vi "gnuplot_legend.vi"(1 "Plot style":i32[](array[numeric])=[1, 3, 6, 2, 4, 7, 5, 8], 2 "Legend":string[](array[string])) -> (0 "Tex String":string)   [LabVIEW 2010]
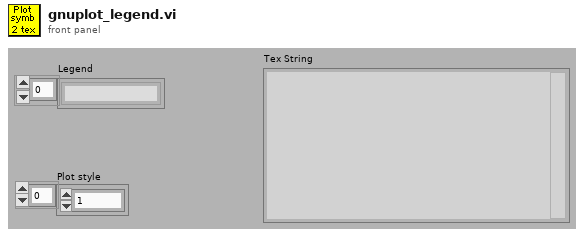
[diagram p1: front panel]
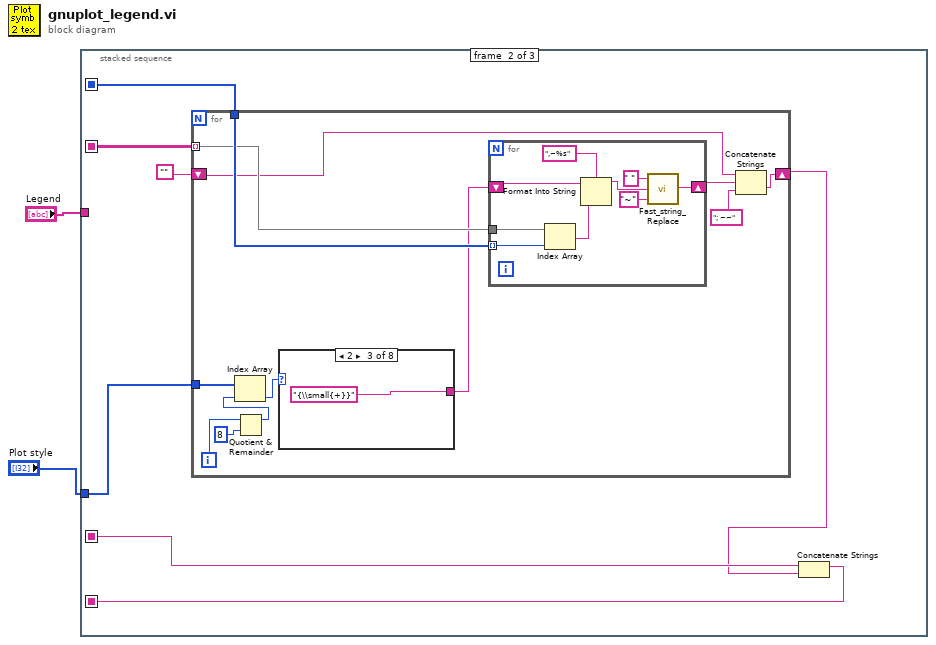
[diagram p0: block diagram]
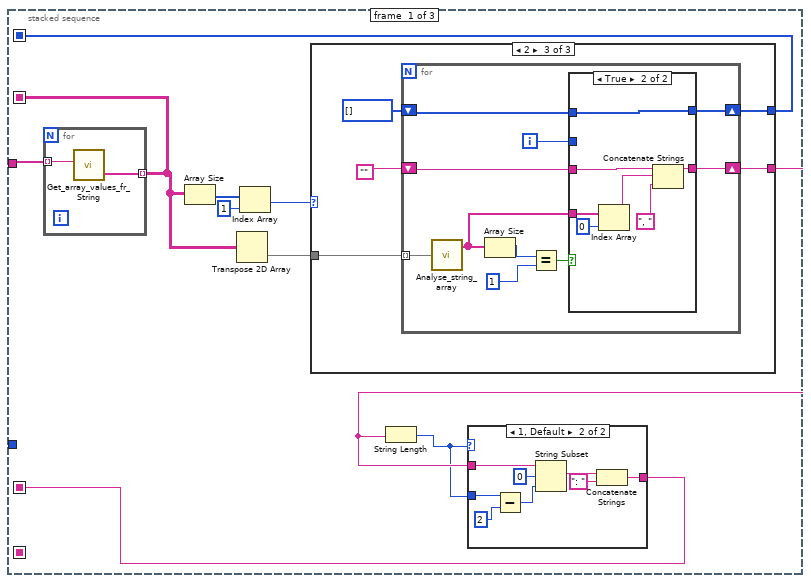
[diagram p2: hidden frame]
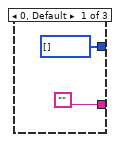
[diagram p4: hidden frame]
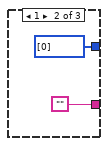
[diagram p5: hidden frame]
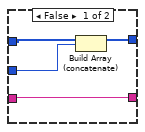
[diagram p6: hidden frame]
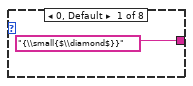
[diagram p7: hidden frame]
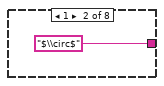
[diagram p8: hidden frame]
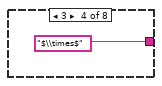
[diagram p9: hidden frame]
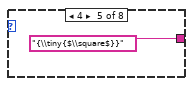
[diagram p10: hidden frame]
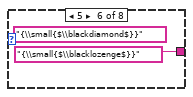
[diagram p11: hidden frame]
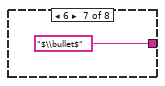
[diagram p12: hidden frame]
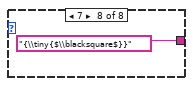
[diagram p13: hidden frame]
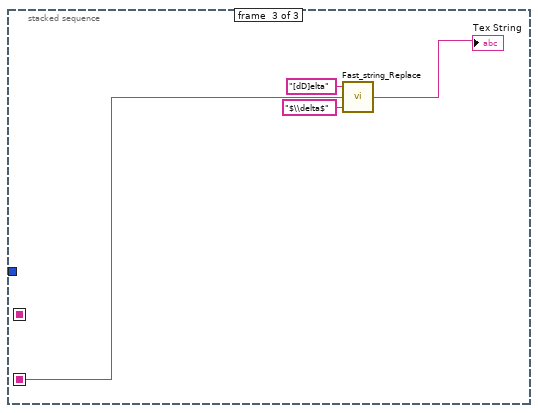
[diagram p14: hidden frame]
diagram:
  n1 = stacked-sequence {
    seq-local: [w8 _ _] -> [_ w60 _]
    seq-local: [w3 _ _] -> [_ w57 _]
    seq-local: [w7 _ _] -> [_ w59 _]
    seq-local: [_ w55 _] -> [_ _ w92]
    tunnel: "Legend" -> [w12 _ _]
    tunnel: "Plot style" -> [_ w54 _]
    frame #0 {
      n2 = for {
        tunnel: w12 -> [w53] mode=indexing
        tunnel: [w52] -> w7 mode=indexing
        n3 = call "Get_array_values_fr_String.vi"("String Value"=w53) -> ("String array"=w52:string[])  [unwired: 1 out]
      }
      n4 = Array Size(array=w7) -> (size(s)=w11:i32[])
      n5 = Transpose 2D Array(2D array=w7) -> (transposed array=w9:string[][])
      n6 = Index Array(array=w11, index=1) -> (element=w6:i32)
      n7 = case shown="2" w6 {
        tunnel: w9 -> [_ _ w30]
        tunnel: [i32[] [] i32[] [0] w28] -> w8
        tunnel: ["" "" w27] -> w5
        frame 0, Default {
        }
        frame 1 {
        }
        frame 2 {
          n8 = for {
            tunnel: w30 -> [w40] mode=indexing
            shift-right: [w34] -> w27
            shift-left: "" -> [w35]
            shift-right: [w32] -> w28
            shift-left: i32[] [] -> [w33]
            i -> [w31]
            n9 = call "Analyse_string_array.vi"("String array"=w40) -> ("Unique strings"=w36:string[])  [unwired: 2 out]
            n10 = Array Size(array=w36) -> (size(s)=w39:i32)
            n11 = Equal?(x=w39, y=1) -> (x = y?=w37:bool)
            n12 = case shown="True" w37 {
              tunnel: w36 -> [_ w51]
              tunnel: w35 -> [w41 w48]
              tunnel: [w41 w47] -> w34
              tunnel: w33 -> [w43 w46]
              tunnel: [w42 w46] -> w32
              tunnel: w31 -> [w44 _]
              frame False {
                n13 = Build Array (concatenate)(w43, w44) -> (w42:i32[])
              }
              frame True {
                n14 = Index Array(array=w51, index=0) -> (element=w49:string)
                n15 = Concatenate Strings(w48, w49, ", " ("string")) -> (w47:string)
              }
            }
          }
        }
      }
      n16 = String Length(string=w5) -> (length=w4:i32)
      n17 = case shown="1, Default" w4 {
        tunnel: w5 -> [w13 w20]
        tunnel: w4 -> [_ w16]
        tunnel: [w13 w17] -> w3
        frame 0 {
        }
        frame 1, Default {
          n18 = Subtract(x=w16, y=2) -> (x-y=w15:i32)
          n19 = String Subset(string=w20, offset (0)=0, length (rest)=w15) -> (substring=w19:string)
          n20 = Concatenate Strings(w19, ": " ("string")) -> (w17:string)
        }
      }
    }
    frame #1 {
      n21 = for {
        tunnel: w60 -> [w72]
        tunnel: w59 -> [w71] mode=indexing
        shift-right: [w69] -> w56
        shift-left: "" -> [w66]
        tunnel: w54 -> [w61]
        i -> [w65]
        n22 = Quotient & Remainder(x=w65, y=8) -> (x-y*floor(x/y)=w63:i32)  [unwired: 1 out]
        n23 = Index Array(array=w61, index=w63) -> (element=w62:i32)
        n24 = case shown="2" w62 {
          tunnel: ["{\\small{$\\diamond$}}" "$\\circ$" "{\\small{+}}" "$\\times$" "{\\tiny{$\\square$}}" "{\\small{$\\blacklozenge$}}" "$\\bullet$" "{\\tiny{$\\blacksquare$}}"] -> w67
          frame 0, Default {
          }
          frame 1 {
          }
          frame 2 {
          }
          frame 3 {
          }
          frame 4 {
          }
          frame 5 {
            (unwired) "{\\small{$\\blackdiamond$}}"
          }
          frame 6 {
          }
          frame 7 {
          }
        }
        n25 = for {
          tunnel: w72 -> [w81] mode=indexing
          tunnel: w71 -> [w80]
          shift-right: [w75] -> w70
          shift-left: w67 -> [w79]
          n26 = Index Array(array=w80, index=w81) -> (element=w78:string)
          n27 = Format Into String(format string=",~%s", initial string=w79, w78) -> (resulting string=w76:string)  [unwired: 1 in, 1 out]
          n28 = call "Fast_string_Replace.vi"("Replace match with:"="~", "Input String"=w76, "regular expression"=" ") -> ("Output String"=w75:string)  [unwired: 2 out]
        }
        n29 = Concatenate Strings(w66, w70, "; ~~" ("string")) -> (w69:string)
      }
      n30 = Concatenate Strings(w57, w56) -> (w55:string)
    }
    frame #2 {
      n31 = call "Fast_string_Replace.vi"("Replace match with:"="$\\delta$", "Input String"=w92, "regular expression"="[dD]elta") -> ("Output String"=→"Tex String":string)  [unwired: 2 out]
    }
  }
